vi "Periodic Tasks.vi"(8 "error in":errorcluster) -> ()   [LabVIEW 2017]
doc: "This VI runs in parallel to other tasks. It can contain as many user-defined periodic loops as you need. These can carry out PID or other sorts of timed response."
uses:
  <vilib>/Rock Robotics/WPI/Utilities/WPI_GetSetVariantRefNum.vi
  Robot Global Data.vi
panel:
  out "Arm Position Global":dbl
  out "Elevator Position Global":dbl
  out "Robot Yaw Global":dbl
  out "Robot Travel Global":dbl format="%#.2f"
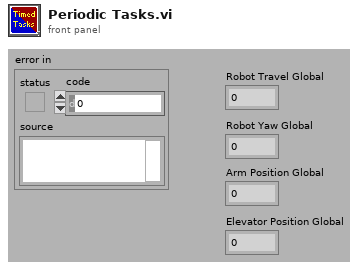
[diagram p1: front panel]
types:
  T1 = typedef "WPI_JoystickDevRef.ctl" = cluster{"Device":T2}
  T2 = typedef "WPI_JoystickDeviceEnum.ctl" = enum16{"USB 0", "USB 1", "USB 2", "USB 3", "USB 4", "USB 5"}
  T3 = typedef "WPI_RobotDriveDevRef.ctl" = cluster{"DevStatus":errorcluster, "Motors[]":T4[], "Square Inputs":bool, "Max Output":dbl}
  T4 = typedef "WPI_MotorControlDeviceRef.ctl" = cluster{"DeviceStatus":errorcluster, "Type":T5, "PWM":cluster{"PWM Channel":T6, "DeadBand":T7}, "CAN":cluster{"Device Number":u8, "SetOutput VI Ref":variant, "GetOutput VI Ref":variant, "Enable VI Ref":variant, "Disable VI Ref":variant, "Data":variant}, "Invert":bool, "DIO PWM":cluster{"PWM \"Enable\" Channel":T6, "DIOChannel":T8, "PWM Rate":dbl}}
  T5 = typedef "WPI_MotorControlType.ctl" = enum16{"PWM", "CAN", "DIO PWM"}
  T6 = typedef "FPGA_DIOPWMChannel.ctl" = enum8{"PWM 0", "PWM 1", "PWM 2", "PWM 3", "PWM 4", "PWM 5", "PWM 6", "PWM 7", "PWM 8", "PWM 9", "PWM MXP 0", "PWM MXP 1", "PWM MXP 2", "PWM MXP 3", "PWM MXP 4", "PWM MXP 5", "PWM MXP 6", "PWM MXP 7", "PWM MXP 8", "PWM MXP 9", "Invalid"}
  T7 = typedef "WPI_PWMDeadband.ctl" = cluster{"Name":string, "maxPositivePwm":i32, "minPositivePwm":i32, "centerPwm":i32, "maxNegativePwm":i32, "minNegativePwm":i32, "angularRange":u16}
  T8 = typedef "FPGA_DIOChannel.ctl" = enum8{"DIO 0", "DIO 1", "DIO 2", "DIO 3", "DIO 4", "DIO 5", "DIO 6", "DIO 7", "DIO 8", "DIO 9", "DIO MXP 0", "DIO MXP 1", "DIO MXP 2", "DIO MXP 3", "DIO MXP 4", "DIO MXP 5", "DIO MXP 6", "DIO MXP 7", "DIO MXP 8", "DIO MXP 9", "DIO MXP 10", "DIO MXP 11", "DIO MXP 12", "DIO MXP 13", "DIO MXP 14", "DIO MXP 15", "SPI Port CS1", "SPI Port CS2", "SPI Port CS3", "SPI Port MISO", "SPI Port MOSI", "Invalid"}
  T9 = cluster{"JoystickDevRef":T1, "RobotDriveDevRef":T3}
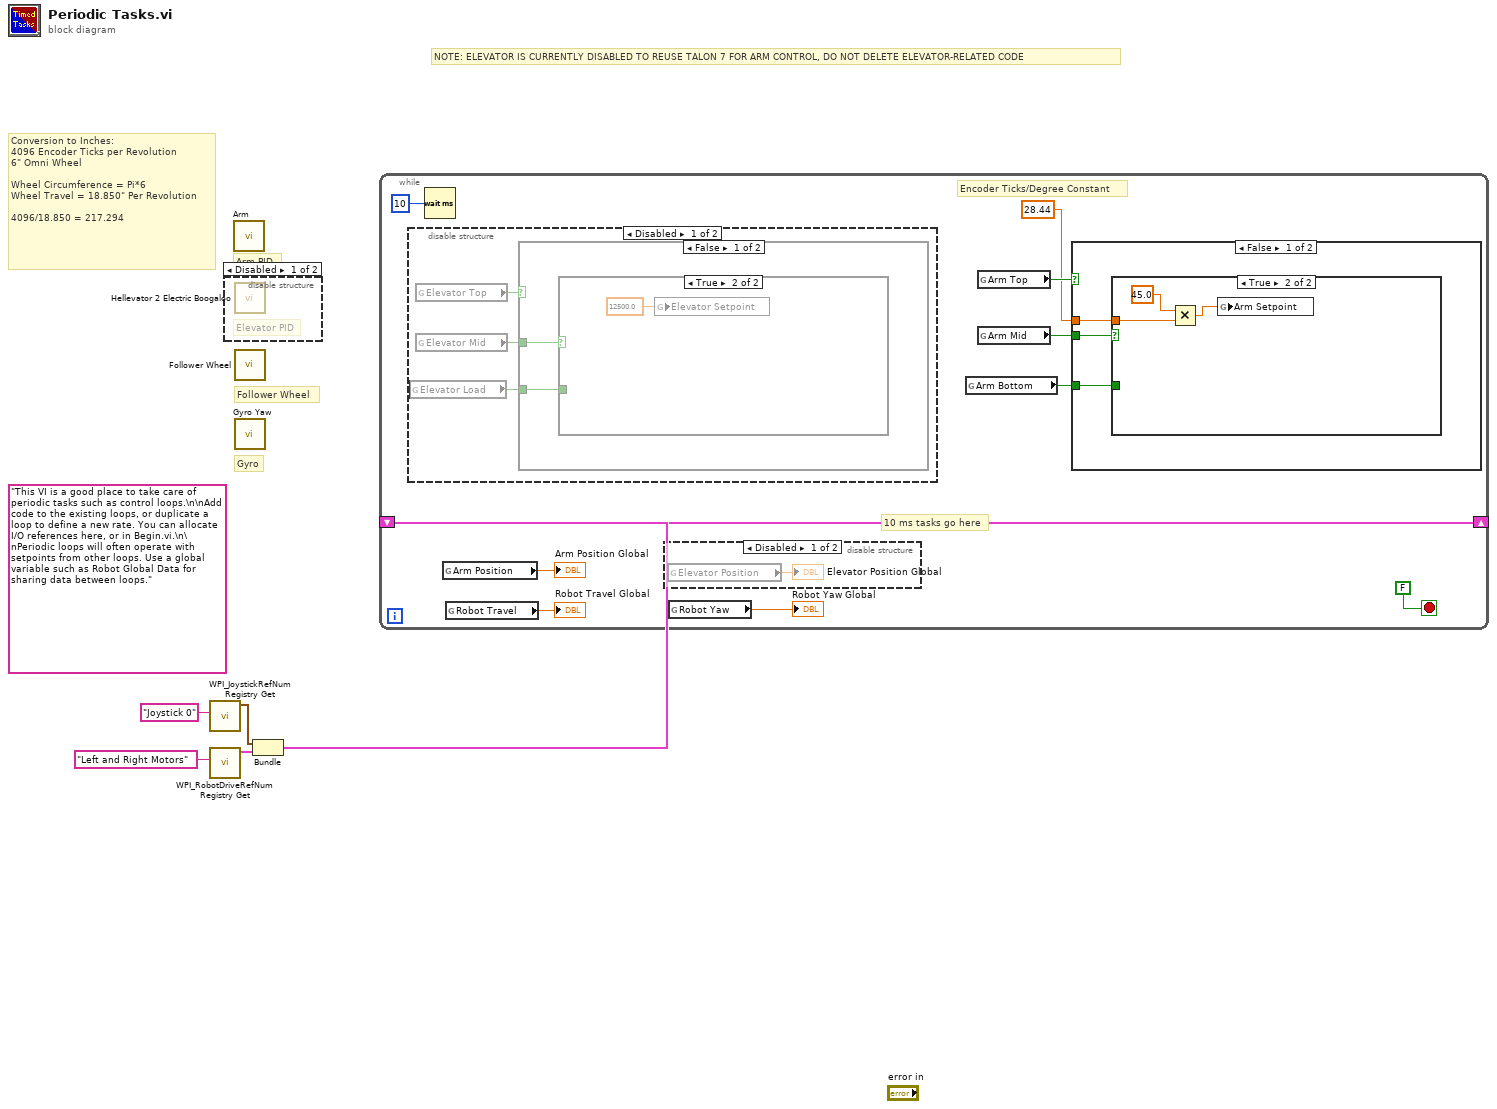
[diagram p0: block diagram]
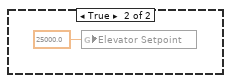
[diagram p5: hidden frame]
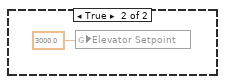
[diagram p6: hidden frame]
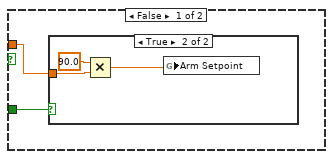
[diagram p8: hidden frame]
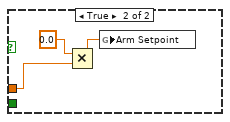
[diagram p10: hidden frame]
diagram:
  (unwired) "This VI is a good place to take care of periodic tasks such as control loops.\n\nAdd code to the existing loops, or duplicate a loop to define a new rate. You can allocate I/O references here, or in Begin.vi.\n\nPeriodic loops will often operate with setpoints from other loops. Use a global variable such as Robot Global Data for sharing data between loops."
  # "NOTE: ELEVATOR IS CURRENTLY DISABLED TO REUSE TALON 7 FOR ARM CONTROL, DO NOT DELETE ELEVATOR-RELATED CODE"
  # "Arm PID"
  # "Gyro"
  # "Follower Wheel"
  # "Conversion to Inches:\n4096 Encoder Ticks per Revolution\n6\" Omni Wheel\n\nWheel Circumference = Pi*6\nWheel Travel = 18.850\" Per Revolution \n\n4096/18.850 = 217.294"
  n1 = call <vilib>:"WPI_JoystickRefNum Registry Get.vi"("refnum name"="Joystick 0") -> ("JoystickDevRef"=w2:T1)  [unwired: 1 in, 9 out]
  n2 = call <vilib>:"WPI_RobotDriveRefNum Registry Get.vi"("refnum name"="Left and Right Motors") -> ("RobotDriveDevRef"=w1:T3)  [unwired: 1 in, 9 out]
  n3 = disable-structure shown="Disabled" {
    frame Disabled {
      # "Elevator PID"
      n4 = call "Hellevator 2 Electric Boogaloo.vi"() -> ()  [unwired: 11 in, 1 out]
    }
    frame Enabled {
    }
  }
  n5 = call "Arm.vi"() -> ()  [unwired: 12 in]
  n6 = call "Follower Wheel.vi"() -> ()  [unwired: 15 in, 1 out]
  n7 = call "Gyro Yaw.vi"() -> ()  [unwired: 12 in]
  n8 = Bundle("JoystickDevRef"=w2, "RobotDriveDevRef"=w1) -> (w5:T9)  [unwired: 1 out]
  n9 = while {
    shift-right: [w13] -> _
    shift-left: w5 -> [w13]
    stop <- FALSE stop-if-true
    # "Encoder Ticks/Degree Constant"
    # "10 ms tasks go here"
    n10 = disable-structure shown="Disabled" {
      frame Disabled {
        n11 = global read "Robot Global Data.vi" "Elevator Load"() -> (w19:bool)
        n12 = global read "Robot Global Data.vi" "Elevator Top"() -> (w17:bool)
        n13 = global read "Robot Global Data.vi" "Elevator Mid"() -> (w18:bool)
        n14 = case shown="False" w17 {
          tunnel: w19 -> [w21 _]
          tunnel: w18 -> [w20 _]
          frame False {
            n15 = case shown="True" w20 {
              tunnel: w21 -> [w22 _]
              frame False {
                n16 = case shown="False" w22 {
                  frame False {
                  }
                  frame True {
                    n17 = global write "Robot Global Data.vi" "Elevator Setpoint"(25000.0 ("Elevator Setpoint")) -> ()
                  }
                }
              }
              frame True {
                n18 = global write "Robot Global Data.vi" "Elevator Setpoint"(12500.0 ("Elevator Setpoint")) -> ()
              }
            }
          }
          frame True {
            n19 = global write "Robot Global Data.vi" "Elevator Setpoint"(3000.0 ("Elevator Setpoint")) -> ()
          }
        }
      }
      frame Enabled {
      }
    }
    n20 = Wait (ms)(milliseconds to wait=u32 10) -> ()  [unwired: 1 out]
    n21 = global read "Robot Global Data.vi" "Arm Position"() -> (→"Arm Position Global":dbl)
    n22 = global read "Robot Global Data.vi" "Robot Travel"() -> (→"Robot Travel Global":dbl)
    n23 = disable-structure shown="Disabled" {
      frame Disabled {
        n24 = global read "Robot Global Data.vi" "Elevator Position"() -> (→"Elevator Position Global":dbl)
      }
      frame Enabled {
      }
    }
    n25 = global read "Robot Global Data.vi" "Robot Yaw"() -> (→"Robot Yaw Global":dbl)
    n26 = global read "Robot Global Data.vi" "Arm Bottom"() -> (w9:bool)
    n27 = global read "Robot Global Data.vi" "Arm Top"() -> (w7:bool)
    n28 = global read "Robot Global Data.vi" "Arm Mid"() -> (w8:bool)
    n29 = case shown="False" w7 {
      tunnel: w9 -> [w28 _]
      tunnel: w8 -> [w27 _]
      tunnel: 28.44 -> [w26 w37]
      frame False {
        n30 = case shown="True" w27 {
          tunnel: w28 -> [w30 _]
          tunnel: w26 -> [w29 w34]
          frame False {
            n31 = case shown="True" w30 {
              tunnel: w29 -> [_ w31]
              frame False {
              }
              frame True {
                n32 = Multiply(x=90.0, y=w31) -> (x*y=w33:dbl)
                n33 = global write "Robot Global Data.vi" "Arm Setpoint"(w33) -> ()
              }
            }
          }
          frame True {
            n34 = Multiply(x=45.0 ("Elevator Setpoint"), y=w34) -> (x*y=w35:dbl)
            n35 = global write "Robot Global Data.vi" "Arm Setpoint"(w35) -> ()
          }
        }
      }
      frame True {
        n36 = Multiply(x=0.0 ("Elevator Setpoint"), y=w37) -> (x*y=w38:dbl)
        n37 = global write "Robot Global Data.vi" "Arm Setpoint"(w38) -> ()
      }
    }
  }
